vi "Configure.vi"(8 "error in":errorcluster, 10 "name":string="CRDS", 11 "eCRDS in":refnum<class "eCRDS.lvclass">) -> (0 "error out":errorcluster, 3 "eCRDS out":refnum<class "eCRDS.lvclass">)   [LabVIEW 2014, in "eCRDS Library.lvlib" / "eCRDS.lvclass"]
doc: "Configures the CRDS for operation and starts all DAQmx tasks associated with the instrument. This VI overrides the parent VI in the Instrument class."
uses:
  eCRDS.lvclass
  Commands/Change Laser Gains/Change Laser Gain CMD.lvclass
  Commands/Change Laser Enable State/Laser Enable CMD.lvclass
  Commands/Change PMT Gains/Change PMT Gain CMD.lvclass
  reusable/Instrument/Instrument.lvclass/Instrument.ctl
  eCRDS.lvclass/eCRDS.ctl
  reusable/Session APIs/File Access/Config Data/Config Data.lvclass/Config Data.ctl
  Commands/Change Laser Gains/Change Laser Gain CMD.lvclass/Change Laser Gain CMD.ctl
  Commands/Change Laser Enable State/Laser Enable CMD.lvclass/Laser Enable CMD.ctl
  Commands/Change PMT Gains/Change PMT Gain CMD.lvclass/Change PMT Gain CMD.ctl
  reusable/Session APIs/File Access/Config Data/Accessors/Read Ref.vi
  reusable/Instrument/Read Log Session.vi
  reusable/Instrument/Read CMD.vi
  reusable/Instrument/Read Cfg Session.vi
  Commands/Change Laser Gains/Write Gains.vi
  Commands/Change Laser Enable State/Write Blue.vi
  Commands/Change Laser Enable State/Write Blue1.vi
  Commands/Change Laser Enable State/Write Red.vi
  Commands/Change PMT Gains/Write Gains.vi
  reusable/CRDS/Main/Read Cells.vi
  <vilib>/Utility/config.llb/Read Key (Double).vi
  <vilib>/Utility/config.llb/Read Key (Boolean).vi
  <vilib>/Utility/config.llb/Read Key (String).vi
  reusable/CRDS/Main/CRDS.lvclass
  <userlib>/_Session Fwk/Session - Root.lvclass
  reusable/CRDS/Cell/CRDS Cell.lvclass
  reusable/Command/Command.lvclass
  reusable/Session APIs/File Access/Config Data/Config Data.lvclass
  reusable/Session APIs/Session Log/System Log.lvclass
  <vilib>/Utility/config.llb/NI_LVConfig.lvlib
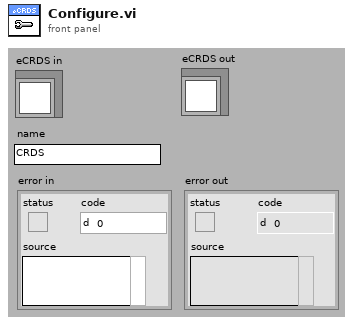
[diagram p1: front panel]
types:
  T1 = cluster{"T (degC)":dbl, "P (mb)":dbl, "Q (lpm)":dbl}
  T2 = typedef "Session - Root.lvclass/Session Handle.ctl" = refnum<data-value>
  T3 = typedef "Config Data.lvclass/Config Session.ctl" = refnum<data-value>
  T4 = cluster{"T (degC)":dbl, "P (mb)":dbl, "Q (lpm)":dbl}[]
  T5 = typedef "NI_LVConfig.lvlib/Config Data RefNum.ctl" = refnum<k1>
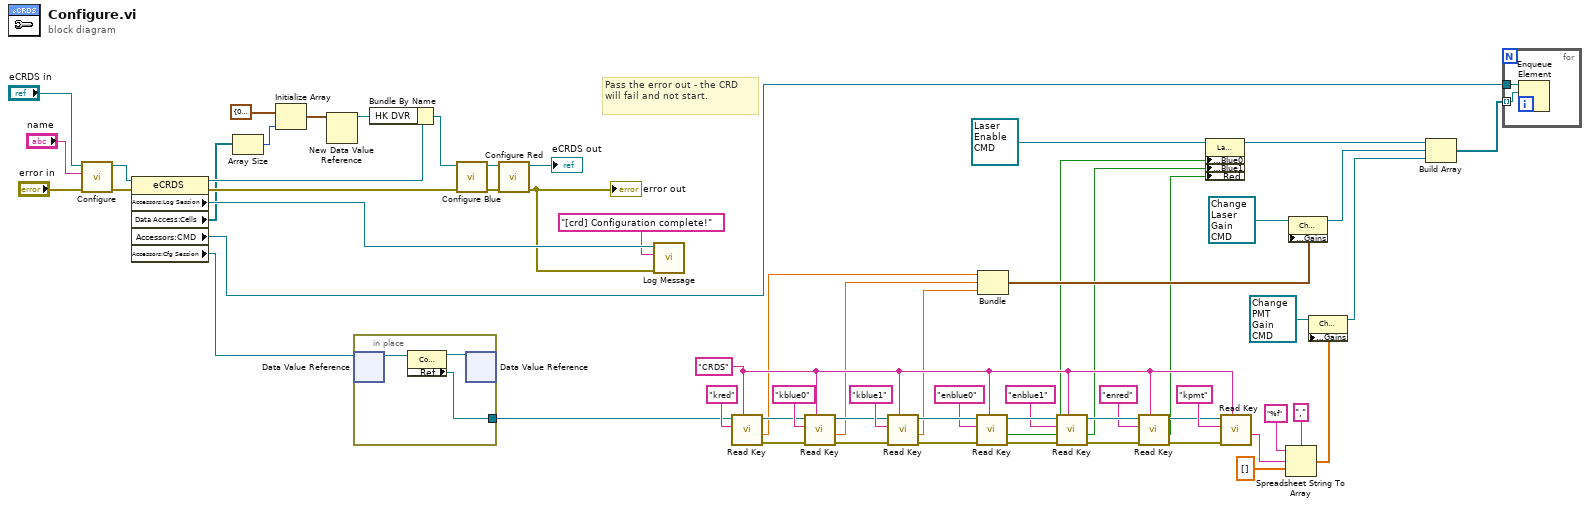
[diagram p0: block diagram]
diagram:
  w19 = "CRDS" ("section")
  # "Pass the error out - the CRD will fail and not start."
  n1 = call-parent "Configure.vi"("error in"="error in", "name"="name", "CRDS in"="eCRDS in") -> ("error out"=w54:errorcluster, "CRDS out"=w58:refnum<class "eCRDS.lvclass">)  [unwired: 7 in]
  n2 = property class="eCRDS"(reference=w58, error in=w54) -> (reference out=w53:refnum<class "eCRDS.lvclass">, error out=w56:errorcluster, "Accessors:Log Session"=w49:T2, "Data Access:Cells"=w45:refnum<class "CRDS Cell.lvclass">[], "Accessors:CMD"=w8:refnum<queue>, "Accessors:Cfg Session"=w1:T3)
  n3 = Array Size(array=w45) -> (size(s)=w44:i32)
  n4 = Initialize Array(T1 {"T (degC)"=0.0, "P (mb)"=0.0, "Q (lpm)"=0.0} ("HK Data"), w44) -> (w43:T4)
  n5 = New Data Value Reference(data value=w43) -> (data value reference=w52:refnum<data-value>)  [unwired: 1 in, 1 out]
  n6 = in-place {
    in-place-border: [w62] -> w18
    n7 = in-place-dvr #1(w1) -> (w64:refnum<class "Config Data.lvclass">)  [unwired: 1 out]
    n8 = property class="Config Data"(reference=w64) -> (reference out=w63:refnum<class "Config Data.lvclass">, "Accessors:Ref"=w62:T5)  [unwired: 1 in, 1 out]
    n9 = in-place-dvr #1(w63) -> ()  [unwired: 2 out]
  }
  n10 = Bundle By Name(cluster=w53, "HK DVR"=w52) -> (w51:refnum<class "eCRDS.lvclass">)
  n11 = call "Configure Blue.vi"("Error In"=w56, "eCRDS in"=w51) -> ("error out"=w55:errorcluster, "eCRDS out"=w57:refnum<class "eCRDS.lvclass">)  [unwired: 8 in]
  n12 = call "Configure Red.vi"("Error In"=w55, "eCRDS in"=w57) -> ("error out"=w47:errorcluster, "eCRDS out"=→"eCRDS out":refnum<class "eCRDS.lvclass">)  [unwired: 8 in]
  "error out" <- w47
  n13 = call "Log Message.vi"("error in"=w47, "MSG In"="[crd] Configuration complete!", "session in"=w49) -> ()  [unwired: 7 in, 2 out]
  n14 = call-poly <vilib>:"Read Key.vi"("section"=w19, "key"="kred" ("section"), "refnum"=w18) -> ("error out"=w38:errorcluster, "value"=w15:dbl, "refnum out"=w37:T5)  [unwired: 5 in, 1 out]
  n15 = call-poly <vilib>:"Read Key.vi"("section"=w19, "error in (no error)"=w38, "key"="kblue0", "refnum"=w37) -> ("error out"=w40:errorcluster, "value"=w14:dbl, "refnum out"=w39:T5)  [unwired: 4 in, 1 out]
  n16 = call-poly <vilib>:"Read Key.vi"("section"=w19, "error in (no error)"=w40, "key"="kblue1", "refnum"=w39) -> ("error out"=w25:errorcluster, "value"=w13:dbl, "refnum out"=w29:T5)  [unwired: 4 in, 1 out]
  n17 = call-poly <vilib>:"Read Key.vi"("section"=w19, "error in (no error)"=w25, "key"="enblue0", "refnum"=w29) -> ("error out"=w26:errorcluster, "value"=w11:bool, "refnum out"=w30:T5)  [unwired: 4 in, 1 out]
  n18 = Bundle("value"=w15, "value"=w14, "value"=w13) -> (w12:cluster{"value":dbl, "value":dbl, "value":dbl})  [unwired: 1 in]
  n19 = call-poly <vilib>:"Read Key.vi"("section"=w19, "error in (no error)"=w26, "key"="enblue1", "refnum"=w30) -> ("error out"=w27:errorcluster, "value"=w10:bool, "refnum out"=w28:T5)  [unwired: 4 in, 1 out]
  n20 = call-poly <vilib>:"Read Key.vi"("section"=w19, "error in (no error)"=w27, "key"="enred", "refnum"=w28) -> ("error out"=w21:errorcluster, "value"=w9:bool, "refnum out"=w22:T5)  [unwired: 4 in, 1 out]
  n21 = property class="Laser Enable CMD.lvclass"(reference=refnum<class "Laser Enable CMD.lvclass"> refnum ("eCRDS Library.lvlib:Laser Enable CMD.lvclass"), "Accessors:Blue0"=w11, "Accessors:Blue1"=w10, "Accessors:Red"=w9) -> (reference out=w7:refnum<class "Laser Enable CMD.lvclass">)  [unwired: 1 in, 1 out]
  n22 = call-poly <vilib>:"Read Key.vi"("section"=w19, "error in (no error)"=w21, "key"="kpmt" ("section"), "refnum"=w22) -> ("value"=w33:string)  [unwired: 4 in, 3 out]
  n23 = Spreadsheet String To Array(delimiter (Tab)=",", format string="%f", spreadsheet string=w33, array type (2D Dbl)=sgl[] []) -> (array=w4:sgl[])
  n24 = property class="Change Laser Gain CMD"(reference=refnum<class "Change Laser Gain CMD.lvclass"> refnum ("eCRDS Library.lvlib:Change Laser Gain CMD.lvclass"), "Accessors:Gains"=w12) -> (reference out=w6:refnum<class "Change Laser Gain CMD.lvclass">)  [unwired: 1 in, 1 out]
  n25 = property class="Change PMT Gains CMD"(reference=refnum<class "Change PMT Gain CMD.lvclass"> refnum ("eCRDS Library.lvlib:Change PMT Gains CMD"), "Accessors:Gains"=w4) -> (reference out=w3:refnum<class "Change PMT Gain CMD.lvclass">)  [unwired: 1 in, 1 out]
  n26 = Build Array(w7, w6, w3) -> (w2:refnum<class "Command.lvclass">[])
  n27 = for {
    tunnel: w8 -> [w66]
    tunnel: w2 -> [w65] mode=indexing
    n28 = Enqueue Element(queue=w66, element=w65) -> ()  [unwired: 2 in, 3 out]
  }
